vi "calc home work.vi"() -> ()   [LabVIEW 2026]
uses:
  <vilib>/measure/NI_MABase.lvlib
panel:
  out "String":string
  out "Waveform Graph":waveform(dbl)(graph)
  in  "Enum":T1(ring)
  in  "stop":bool
  in  "b":dbl
  in  "a":dbl
  out "o/p":dbl
  # "MY PROJECT"
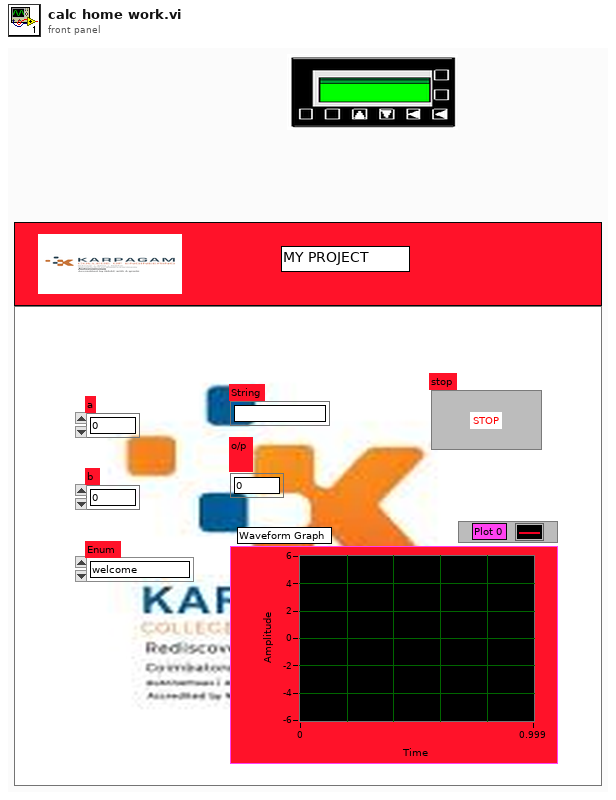
[diagram p1: front panel]
types:
  T1 = enum16{"welcome", "graph", "div", "mul", "sub", "add"}
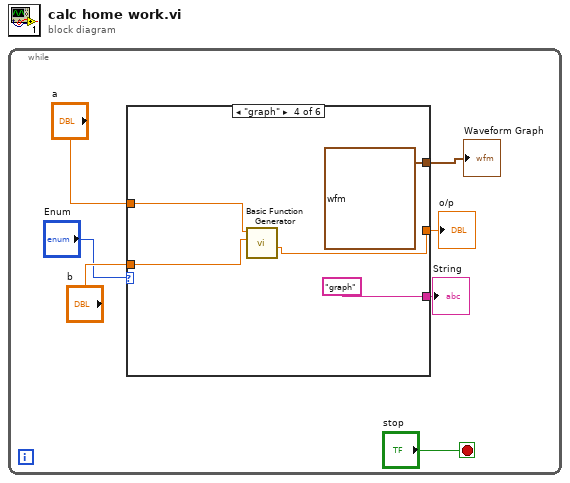
[diagram p0: block diagram]
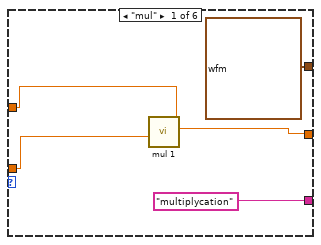
[diagram p2: hidden frame]
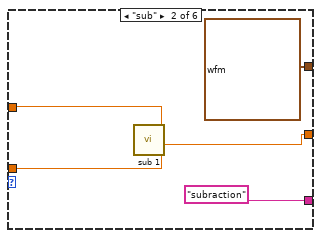
[diagram p3: hidden frame]
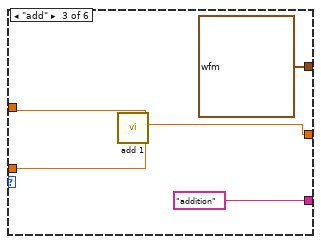
[diagram p4: hidden frame]
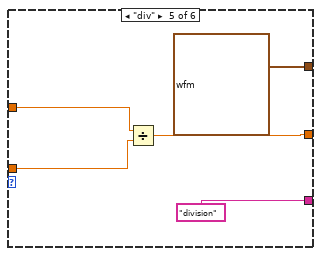
[diagram p5: hidden frame]
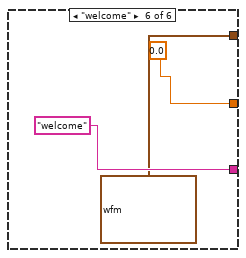
[diagram p6: hidden frame]
diagram:
  n1 = while {
    stop <- "stop" stop-if-true
    n2 = case shown="\"graph\"" "Enum" {
      tunnel: "a" -> [w12 w17 w22 w27 w32 _]
      tunnel: "b" -> [w11 w16 w21 w26 w31 _]
      tunnel: [w10 w15 w20 w25 w30 0.0 ("phase out")] -> w5
      tunnel: ["multiplycation" "subraction" "addition" "graph" "division" "welcome"] -> w2
      tunnel: [waveform(dbl) {"t0"=timestamp(0 s since 1904-01-01), "dt"=1.0, "Y"=[]} ("Waveform Chart") waveform(dbl) {"t0"=timestamp(0 s since 1904-01-01), "dt"=1.0, "Y"=[]} ("Waveform Chart") waveform(dbl) {"t0"=timestamp(0 s since 1904-01-01), "dt"=1.0, "Y"=[]} ("Waveform Chart") waveform(dbl) {"t0"=timestamp(133.0 s since 1904-01-01), "dt"=0.001, "Y"=array[1000 elements]} ("Waveform Chart") waveform(dbl) {"t0"=timestamp(0 s since 1904-01-01), "dt"=1.0, "Y"=[]} ("Waveform Chart") waveform(dbl) {"t0"=timestamp(0 s since 1904-01-01), "dt"=1.0, "Y"=[]} ("Waveform Chart")] -> w1
      frame "mul" {
        n3 = call "mul 1.vi"("y"=w11, "x"=w12) -> ("x*y"=w10:dbl)  [unwired: 9 in]
      }
      frame "sub" {
        n4 = call "sub 1.vi"("Numeric 2"=w16, "Numeric"=w17) -> ("Numeric 3"=w15:dbl)  [unwired: 9 in]
      }
      frame "add" {
        n5 = call "add 1.vi"("Numeric 2"=w21, "Numeric"=w22) -> ("Numeric 3"=w20:dbl)  [unwired: 9 in]
      }
      frame "graph" {
        n6 = call <vilib>:"Basic Function Generator.vi"("amplitude"=w26, "frequency"=w27) -> ("phase out"=w25:dbl)  [unwired: 7 in, 2 out]
      }
      frame "div" {
        n7 = Divide(x=w32, y=w31) -> (x/y=w30:dbl)
      }
      frame "welcome" {
      }
    }
    "o/p" <- w5
    "String" <- w2
    "Waveform Graph" <- w1
  }
